vi "Dielectric Material Properties.vi"(6 "m-nm Dielectric":dbl, 8 "Dielectric Thickness  in":dbl, 9 "Energy (Heat; I^2R)":dbl, 11 "NS Base Area":dbl) -> (0 "Dielectric Specfic Heat Capacity":dbl, 1 "Mass Dielectric":dbl, 2 "Dielectric Density":dbl, 3 "Volume Dielectric":dbl, 4 "Delta Temp Change \nDielectric":dbl, 5 "Dielectric Thickness  out":dbl, 10 "mc":dbl)   [LabVIEW 2020]
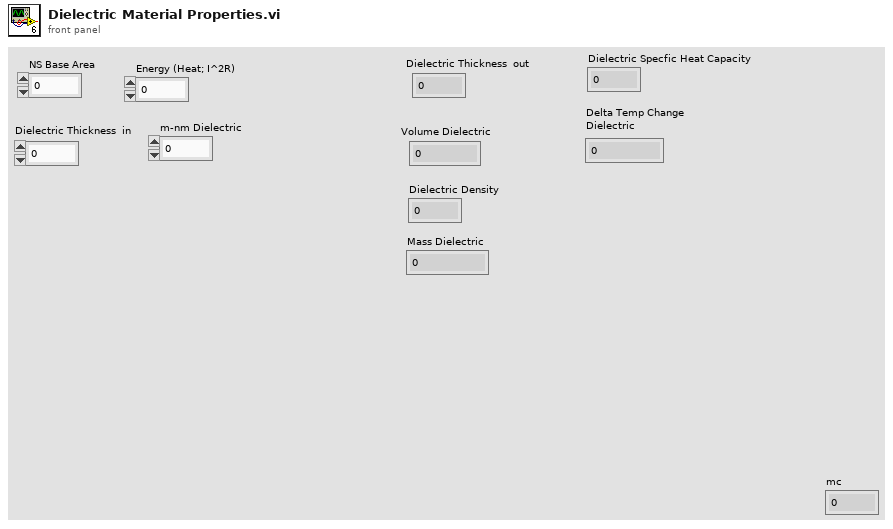
[diagram p1: front panel]
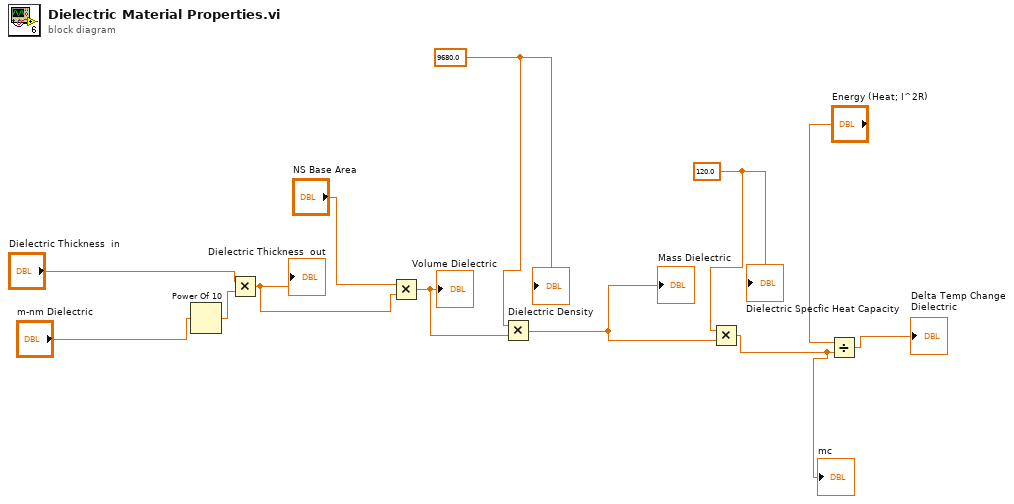
[diagram p0: block diagram]
diagram:
  w2 = 120.0 ("Silicon Specfic Heat Capacity 8")
  w3 = 9680.0 ("Silicon Density 8")
  n1 = Power Of 10(x="m-nm Dielectric") -> (10^x=w4:dbl)
  n2 = Multiply(x="Dielectric Thickness  in", y=w4) -> (x*y=w7:dbl)
  "Dielectric Thickness  out" <- w7
  n3 = Multiply(x="NS Base Area", y=w7) -> (x*y=w8:dbl)
  "Volume Dielectric" <- w8
  n4 = Multiply(x=w3, y=w8) -> (x*y=w12:dbl)
  "Mass Dielectric" <- w12
  n5 = Multiply(x=w2, y=w12) -> (x*y=w1:dbl)
  "mc" <- w1
  n6 = Divide(x="Energy (Heat; I^2R)", y=w1) -> (x/y=→"Delta Temp Change \nDielectric":dbl)
  "Dielectric Density" <- w3
  "Dielectric Specfic Heat Capacity" <- w2
